vi "Drag.vi"(0 "FSM.Edge in":refnum<class "FSM.Edge.lvclass">, 9 "delta":cluster{"X":dbl, "Y":dbl}) -> (4 "FSM.Edge out":refnum<class "FSM.Edge.lvclass">)   [LabVIEW 2020, in "FSM.Edge.lvclass"]
uses:
  FSM.Edge.lvclass
  FSM.Edge.lvclass/FSM.Edge.ctl
  FSM.Label/FSM.Label.lvclass
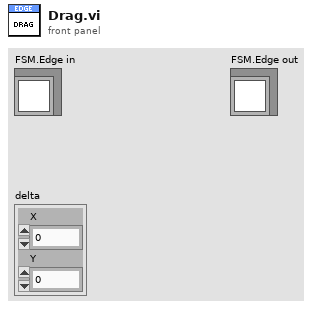
[diagram p1: front panel]
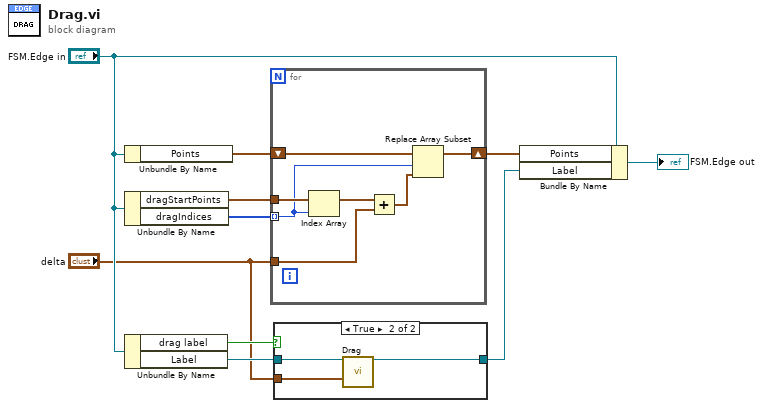
[diagram p0: block diagram]
diagram:
  n1 = Unbundle By Name("FSM.Edge in") -> ("Points"=w9:cluster{"x":i16, "y":i16}[])
  n2 = Unbundle By Name("FSM.Edge in") -> ("dragStartPoints"=w7:cluster{"x":i16, "y":i16}[], "dragIndices"=w6:i32[])
  n3 = Unbundle By Name("FSM.Edge in") -> ("drag label"=w4:bool, "Label"=w2:refnum<class "FSM.Label.lvclass">)
  n4 = for {
    tunnel: "delta" -> [w15]
    shift-right: [w14] -> w8
    shift-left: w9 -> [w17]
    tunnel: w7 -> [w16]
    tunnel: w6 -> [w11] mode=indexing
    n5 = Index Array(array=w16, index=w11) -> (element=w12:cluster{"x":i16, "y":i16})
    n6 = Add(x=w12, y=w15) -> (x+y=w13:cluster{dbl, dbl})
    n7 = Replace Array Subset(array=w17, new element=w13, index=w11) -> (w14:cluster{"x":i16, "y":i16}[])
  }
  n8 = case shown="True" w4 {
    tunnel: [w18 w20] -> w3
    tunnel: w2 -> [w18 w21]
    tunnel: "delta" -> [_ w19]
    frame False {
    }
    frame True {
      n9 = call "Drag.vi"("FSM.Label In"=w21, "delta"=w19) -> ("FSM.Label Out"=w20:refnum<class "FSM.Label.lvclass">)  [unwired: 13 in]
    }
  }
  n10 = Bundle By Name(cluster="FSM.Edge in", "Points"=w8, "Label"=w3) -> (→"FSM.Edge out":refnum<class "FSM.Edge.lvclass">)
